vi "Analys.vi"(8 "error in (no error)":errorcluster, 9 "Data link":variant, 10 "data":T1) -> (0 "error out":errorcluster)   [LabVIEW 2019, in "DOWNLINK.lvlib"]
doc: "Run analys of error on bit\n_____\nCreated using Delacor QMH Event Scripter 4.2.1.88."
uses:
  DOWNLINK.lvlib
  TypeDef/Analys data.ctl
  TypeDef/Analys type.ctl
  Analys Argument--cluster.ctl
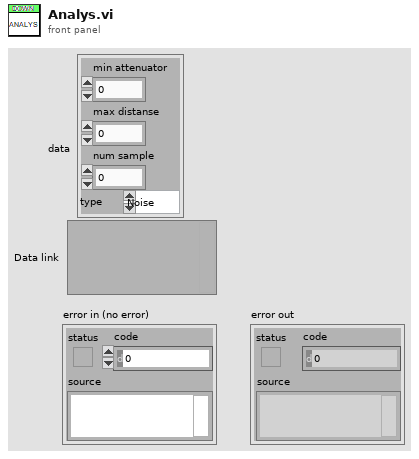
[diagram p1: front panel]
types:
  T1 = typedef "Analys data.ctl" = cluster{"min attenuator":dbl, "max distanse":dbl, "num sample":dbl, "type":T2}
  T2 = typedef "Analys type.ctl" = enum16{"Noise", "Distance"}
  T3 = typedef "DOWNLINK.lvlib/Analys Argument--cluster.ctl" = cluster{"Data link":variant, "data":T1}
  T4 = typedef "DOWNLINK.lvlib/Request Events--cluster.ctl" = cluster{"Stop Module":refnum<user-event>, "Do Something":refnum<user-event>, "Do Something Else":refnum<user-event>, "Do Something Else and Wait for Reply":refnum<user-event>, "Show Panel":refnum<user-event>, "Hide Panel":refnum<user-event>, "Get Module Execution Status":refnum<user-event>, "Show Diagram":refnum<user-event>, "CH_LINK":refnum<user-event>, "Show Power":refnum<user-event>, "Analys":refnum<user-event>}
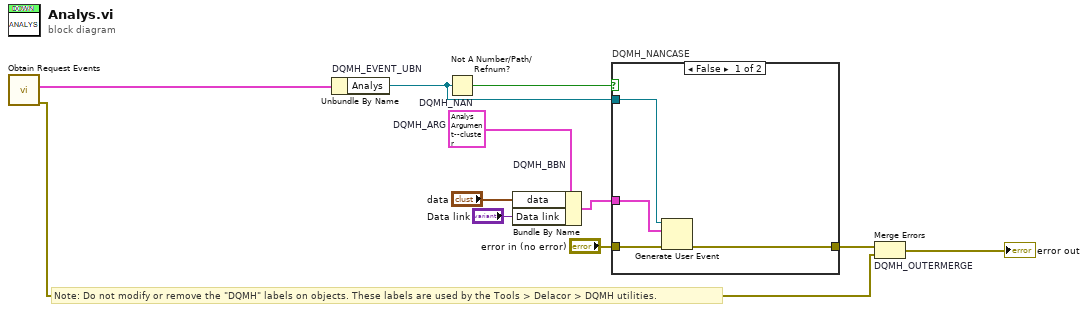
[diagram p0: block diagram]
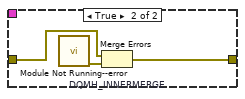
[diagram p2: hidden frame]
diagram:
  w5 = T3 {"Data link"=variant, "data"={"min attenuator"=0.0, "max distanse"=0.0, "num sample"=0.0, "type"=enum."Noise"}}  # DQMH_ARG
  # "Note: Do not modify or remove the \"DQMH\" labels on objects. These labels are used by the Tools > Delacor > DQMH utilities."
  n1 = call "Obtain Request Events.vi"() -> ("error out"=w4:errorcluster, "DOWNLINK Request Events"=w3:T4)  [unwired: 10 in]
  n2 = Unbundle By Name "DQMH_EVENT_UBN"(w3) -> ("Analys"=w7:refnum<user-event>)
  n3 = Not A Number/Path/Refnum? "DQMH_NAN"(number/path/refnum=w7) -> (NaN/Path/Refnum?=w8:bool)
  n4 = Bundle By Name "DQMH_BBN"(cluster=w5, "data"="data", "Data link"="Data link") -> (w9:T3)
  n5 = case "DQMH_NANCASE" shown="False" w8 {
    tunnel: "error in (no error)" -> [w15 w18]
    tunnel: [w14 w17] -> w6
    tunnel: w7 -> [w13 _]
    tunnel: w9 -> [w12 _]
    frame False {
      n6 = Generate User Event(user event=w13, event data cluster=w12, error in=w15) -> (error out=w14:errorcluster)  [unwired: 1 in, 1 out]
    }
    frame True {
      n7 = call "Module Not Running--error.vi"() -> ("error out"=w16:errorcluster)  [unwired: 11 in]
      n8 = Merge Errors "DQMH_INNERMERGE"(w18, w16) -> (w17:errorcluster)
    }
  }
  n9 = Merge Errors "DQMH_OUTERMERGE"(w6, w4) -> (→"error out":errorcluster)
